vi "Save Test Report.vi"(8 "error in (no error)":errorcluster, 10 "Result Actor.lvlib:Results.lvclass":refnum<class "Results.lvclass">, 11 "SystemLink Logger in":refnum<class "SystemLink Logger.lvclass">) -> (0 "error out":errorcluster, 3 "SystemLink Logger out":refnum<class "SystemLink Logger.lvclass">)   [LabVIEW 2016, in "Logging.lvlib" / "SystemLink Logger.lvclass"]
uses:
  SystemLink Logger.lvclass
  Results/Results.lvclass
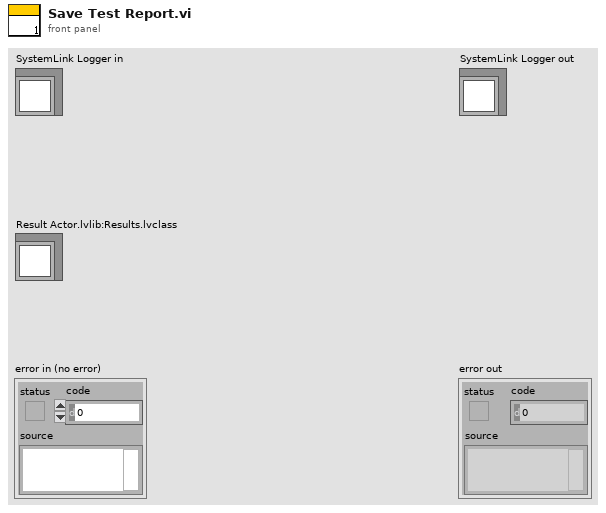
[diagram p1: front panel]
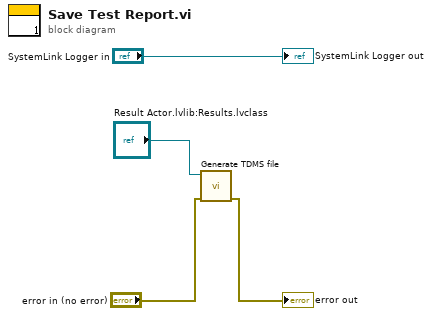
[diagram p0: block diagram]
diagram:
  n1 = call-dynamic "Generate TDMS file.vi"("error in (no error)"="error in (no error)", "Results in"="Result Actor.lvlib:Results.lvclass") -> ("error out"=→"error out":errorcluster)  [unwired: 7 in, 2 out]
  "SystemLink Logger out" <- "SystemLink Logger in"
